vi "Update Chat[ ].vi"(8 "error in (no error)":errorcluster, 10 "Message":variant, 11 "Telegram Class in":refnum<class "Telegram Class.lvclass">) -> (0 "error out":errorcluster, 3 "Telegram Class out":refnum<class "Telegram Class.lvclass">)   [LabVIEW 2015, in "Telegram Library.lvlib" / "Telegram Class.lvclass"]
doc: "Created IvanLis by LabVIEW Portal\nProfile: http://labviewportal.org/memberlist.php?mode=viewprofile&u=987\neMail: IvanLisanov@gMail.com\nTelegram: https://t.me/IvanLis"
uses:
  Telegram Class.lvclass
  JSON Library/TypeDef/Chat.ctl
  TypeDef/Chat.ctl
  Telegram Class.lvclass/Telegram Class.ctl
  JSON Library/JSON Library.lvlib
  Telegram Library.lvlib
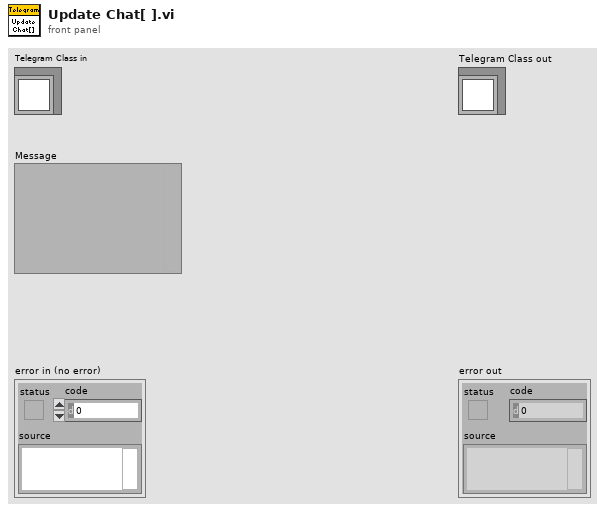
[diagram p1: front panel]
types:
  T1 = typedef "JSON Library.lvlib/Chat.ctl" = cluster{"@type":string, "id":i64, "title":string}
  T2 = typedef "Telegram Library.lvlib/Chat.ctl" = cluster{"id":i64, "position":i64, "title":string}
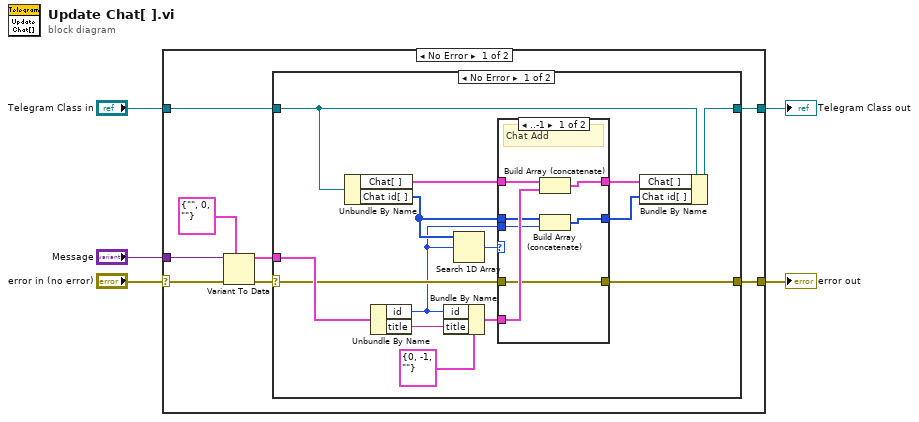
[diagram p0: block diagram]
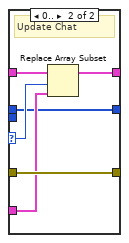
[diagram p2: hidden frame]
diagram:
  n1 = case shown="No Error" "error in (no error)" {
    selector: "error in (no error)" -> [w13 w44]
    tunnel: [w8 w44] -> w4
    tunnel: [w6 w43] -> w2
    tunnel: "Telegram Class in" -> [w7 w43]
    tunnel: "Message" -> [w11 _]
    frame No Error {
      n2 = Variant To Data(error in=w13, type=T1 {"@type"="", "id"=0, "title"=""} ("Message"), Variant=w11) -> (data=w10:T1, error out=w9:errorcluster)
      n3 = case shown="No Error" w9 {
        selector: w9 -> [w21 w42]
        tunnel: w10 -> [w27 _]
        tunnel: [w24 w42] -> w8
        tunnel: w7 -> [w25 w41]
        tunnel: [w19 w41] -> w6
        frame No Error {
          n4 = Unbundle By Name(w25) -> ("Chat[ ]"=w20:T2[], "Chat id[ ]"=w16:i64[])
          n5 = Unbundle By Name(w27) -> ("id"=w14:i64, "title"=w17:string)
          n6 = Bundle By Name(cluster=T2 {"id"=0, "position"=-1, "title"=""} ("Chat"), "id"=w14, "title"=w17) -> (w26:T2)
          n7 = Search 1D Array(1D array=w16, element=w14) -> (index of element=w22:i32)  [unwired: 1 in]
          n8 = case shown="..-1" w22 {
            selector: w22 -> [_ w37]
            tunnel: w21 -> [w31 w40]
            tunnel: w26 -> [w32 w36]
            tunnel: [w31 w40] -> w24
            tunnel: w20 -> [w34 w39]
            tunnel: [w33 w38] -> w18
            tunnel: w16 -> [w30 w35]
            tunnel: [w29 w35] -> w15
            tunnel: w14 -> [w28 _]
            frame ..-1 {
              # "Chat Add"
              n9 = Build Array (concatenate)(w34, w32) -> (w33:T2[])
              n10 = Build Array (concatenate)(w30, w28) -> (w29:i64[])
            }
            frame 0.. {
              # "Update Chat"
              n11 = Replace Array Subset(array=w39, new element=w36, index=w37) -> (w38:T2[])
            }
          }
          n12 = Bundle By Name(cluster=w25, "Chat[ ]"=w18, "Chat id[ ]"=w15) -> (w19:refnum<class "Telegram Class.lvclass">)
        }
        frame Error {
        }
      }
    }
    frame Error {
    }
  }
  "error out" <- w4
  "Telegram Class out" <- w2
